vi "Close.vi"(8 "error in (no error)":errorcluster, 11 "Modbus in":refnum<class "Modbus.lvclass">) -> (0 "error out":errorcluster, 3 "Modbus out":refnum<class "Modbus.lvclass">)   [LabVIEW 2018, in "Modbus.lvclass"]
doc: "Modbus.lvclass:Close.vi\n\nThis VI closes the Modbus resources..\n\nInstrument Communication Module Version 1.0\nJanuary, 2017 Original Code Consulting David Thomson\n www.originalcode.com"
uses:
  Modbus.lvclass
  Modbus.lvclass/Modbus.ctl
  <vilib>/Modbus/master/Modbus Master.lvclass
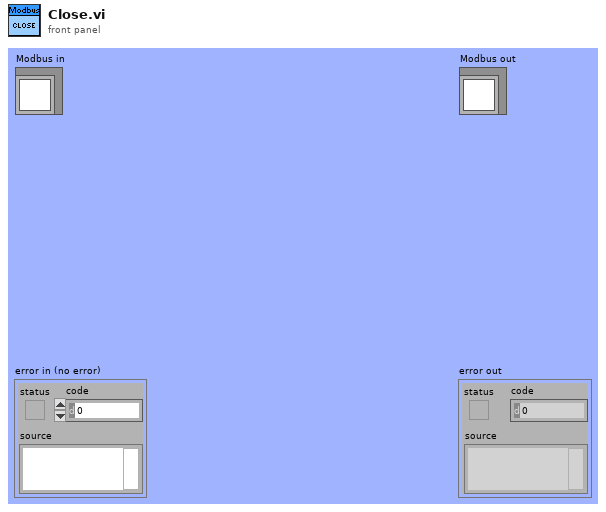
[diagram p1: front panel]
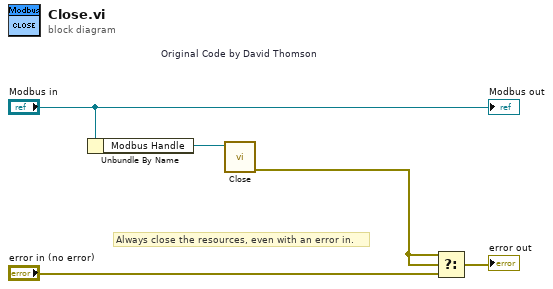
[diagram p0: block diagram]
diagram:
  # "Always close the resources, even with an error in."
  n1 = Unbundle By Name "Original Code by David Thomson"("Modbus in") -> ("Modbus Handle"=w2:refnum<class "Modbus Master.lvclass">)
  n2 = call-dynamic "Close.vi"("Modbus master in"=w2) -> ("error out"=w3:errorcluster)  [unwired: 10 in]
  n3 = Select(t=w3, s=w3, f="error in (no error)") -> (s? t:f=→"error out":errorcluster)
  "Modbus out" <- "Modbus in"
